vi "Feature Name.vi"() -> (2 "Feature name":string, 3 "Out":bool)   [LabVIEW 2015]
uses:
  Control Button/Exit.ctl
  Control PB/Next_.ctl
panel:
  in  "Feature list":string="Ionizer"
  in  "Next":T1
  in  "Exit":T2
  # "Add Feature List"
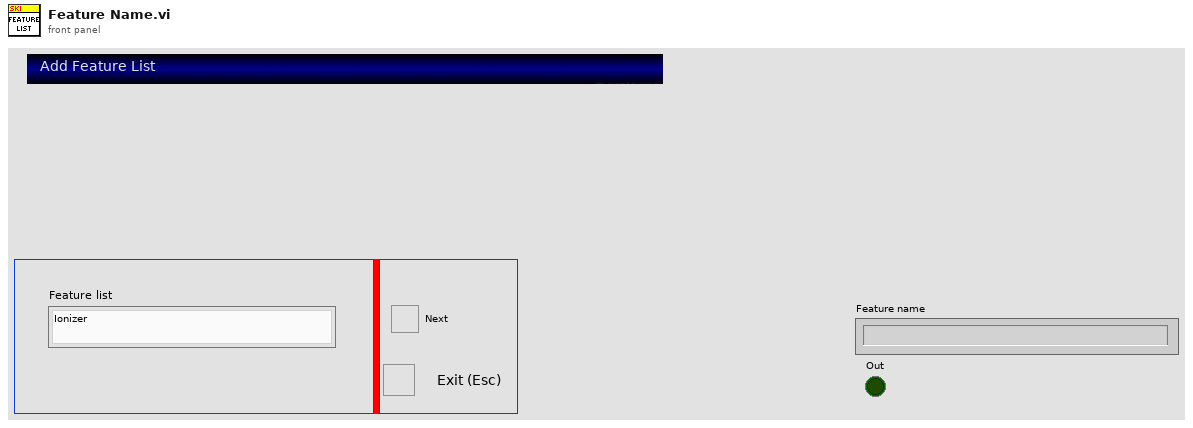
[diagram p1: front panel]
types:
  T1 = typedef "Next_.ctl" = bool
  T2 = typedef "Exit.ctl" = bool
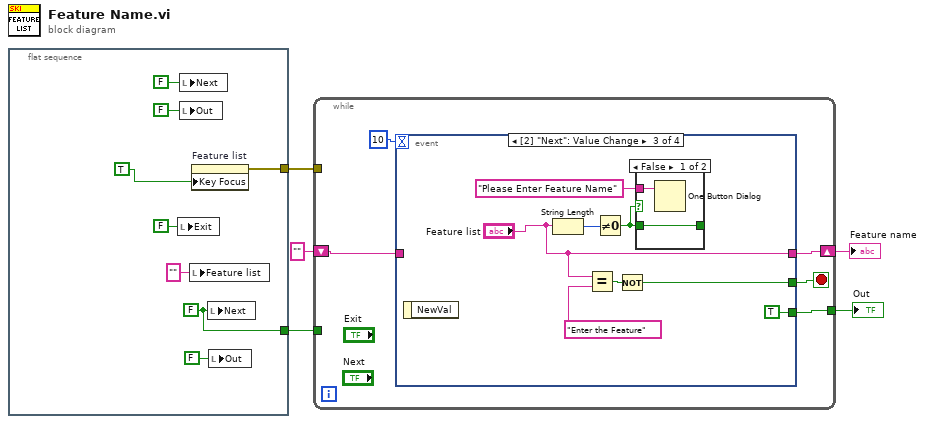
[diagram p0: block diagram]
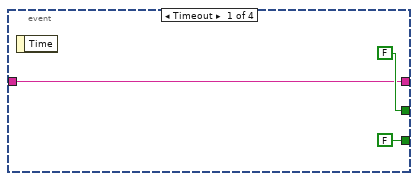
[diagram p2: hidden frame]
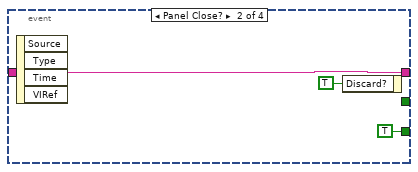
[diagram p3: hidden frame]
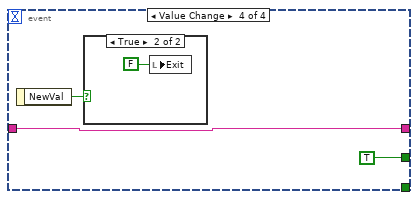
[diagram p5: hidden frame]
diagram:
  n1 = flat-sequence {
    tunnel: [w10] -> w3
    tunnel: [w7] -> w2
    frame #0 {
      w10 = T1 FALSE ("Next")
      n2 = local write "Exit"(FALSE ("Exit")) -> ()
      n3 = local write "Next"(T1 FALSE ("Next")) -> ()
      n4 = local write "Out"(FALSE ("Out")) -> ()
      n5 = local write "Feature list"("" ("Feature list")) -> ()
      n6 = property on="Feature list" class="Str"("Key Focus"=TRUE) -> (error out=w7:errorcluster)  [unwired: 2 in, 1 out]
      n7 = local write "Next"(w10) -> ()
      n8 = local write "Out"(FALSE ("Out")) -> ()
    }
  }
  n9 = while {
    tunnel: [w16] -> w4
    tunnel: w3 -> [_]
    shift-right: [w17] -> w5
    shift-left: "" ("Feature list") -> [w14]
    tunnel: w2 -> [_]
    stop <- w18 stop-if-true
    n10 = event shown="[2] \"Next\": Value Change" {
      selector: _ -> [_ _ _ _]
      dyn-events: _ -> [_ _ _ _]
      timeout: 10 -> [_ _ _ _]
      tunnel: [FALSE _ w27 TRUE] -> w18
      tunnel: [w19 w22 "Feature list" w36] -> w17
      tunnel: [T1 FALSE ("NewVal") T1 TRUE ("NewVal") T1 TRUE ("NewVal") _] -> w16
      tunnel: w14 -> [w19 w22 _ w36]
      event Timeout {
        n11 = event-data() -> ()  [unwired: 1 in, 1 out]
      }
      event Panel Close? {
        n12 = event-data() -> ()  [unwired: 1 in, 4 out]
        n13 = event-data("Discard?"=TRUE) -> ()  [unwired: 1 in, 1 out]
      }
      event Value Change {
        n14 = event-data() -> ()  [unwired: 1 in, 1 out]
        n15 = String Length(string="Feature list") -> (length=w32:i32)
        n16 = Equal?(x="Feature list", y="Enter the Feature") -> (x = y?=w28:bool)
        n17 = Not Equal To 0?(x=w32) -> (x != 0?=w30:bool)
        n18 = Not(x=w28) -> (.not. x?=w27:bool)
        n19 = case shown="False" w30 {
          tunnel: "Please Enter Feature Name" ("message") -> [w34 _]
          tunnel: [w33 w35] -> _
          tunnel: w30 -> [w33 w35]
          frame False {
            n20 = One Button Dialog(message=w34) -> ()  [unwired: 1 in, 1 out]
          }
          frame True {
          }
        }
      }
      event Value Change {
        n21 = event-data() -> ("NewVal"=w37:T2)  [unwired: 1 in]
        n22 = case shown="True" w37 {
          frame False {
          }
          frame True {
            n23 = local write "Exit"(T1 FALSE ("Next")) -> ()
          }
        }
      }
    }
  }
  "Feature name" <- w5
  "Out" <- w4
